vi "Agilent 6000 Series Acquire Waveform.vi"() -> ()   [LabVIEW 2017]
doc: "This example shows how to use autosetup and acquire a waveform on a single channel."
uses:
  <instrlib>/Agilent 6000 Series/Public/Data/Read Single Waveform.vi
  <instrlib>/Agilent 6000 Series/Agilent 6000 Series.lvlib
panel:
  in  "Source (0: Channel 1)":u16(ring) items=["Channel 1", "Channel 2", "Channel 3", "Channel 4", "Math"]
  in  "Probe Attenuation (1.0)":dbl=1.0
  in  "Timeout (10000 ms)":u32=10000
  out "Waveform Data":waveform(dbl)(graph)
  in  "VISA resource name":refnum<visa-resource-name>
  # "(c) 2009-2015 National Instruments.  ALL RIGHTS RESERVED."
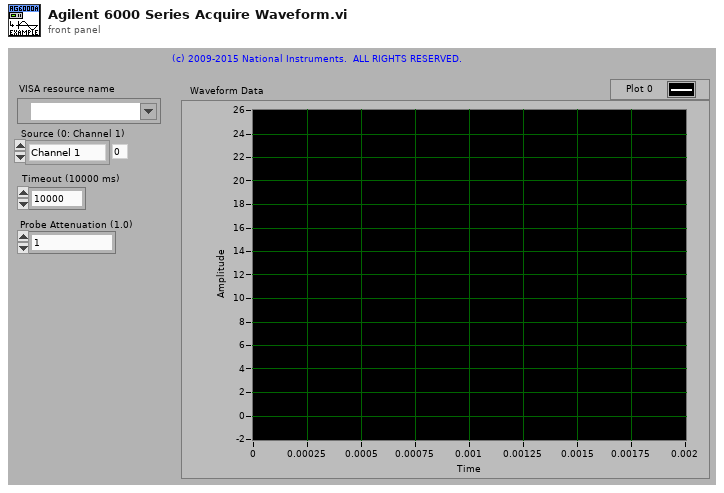
[diagram p1: front panel]
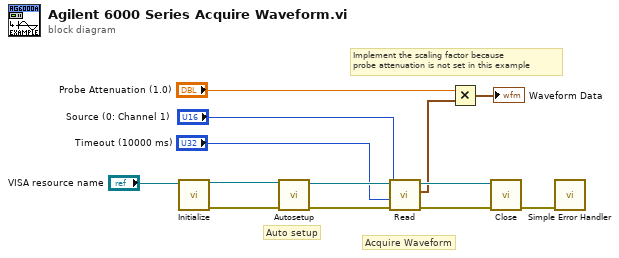
[diagram p0: block diagram]
diagram:
  # "Implement the scaling factor because\nprobe attenuation is not set in this example"
  # "Acquire Waveform"
  # "Auto setup"
  n1 = call <instrlib>:"Initialize.vi"("VISA resource name"="VISA resource name") -> ("error out"=w9:errorcluster, "VISA resource name out"=w8:refnum<visa-resource-name>)  [unwired: 9 in]
  n2 = call <instrlib>:"Autosetup.vi"("error in (no error)"=w9, "VISA resource name"=w8) -> ("error out"=w6:errorcluster, "VISA resource name out"=w7:refnum<visa-resource-name>)  [unwired: 8 in]
  n3 = call-poly <instrlib>:"Read.vi"("error in (no error)"=w6, "Timeout (10000 ms)"="Timeout (10000 ms)", "Source (0: Channel 1)"="Source (0: Channel 1)", "VISA resource name"=w7) -> ("error out"=w11:errorcluster, "Waveform Data"=w3:waveform(dbl), "VISA resource name out"=w12:refnum<visa-resource-name>)  [unwired: 5 in]
  n4 = Multiply(x="Probe Attenuation (1.0)", y=w3) -> (x*y=→"Waveform Data":waveform(dbl))
  n5 = call <instrlib>:"Close.vi"("error in (no error)"=w11, "VISA resource name"=w12) -> ("error out"=w13:errorcluster)  [unwired: 9 in]
  n6 = call <vilib>:"Simple Error Handler.vi"("error in (no error)"=w13) -> ()  [unwired: 4 in, 5 out]
